vi "User - Filter List.vi"(8 "Error In":errorcluster, 9 "Data to Search":string[](array[string]), 10 "Search From":string[](array[string]), 11 "All List":string[](array[string])) -> (0 "Error Out":errorcluster, 3 "Data Out":string[](array[string]))   [LabVIEW 2020]
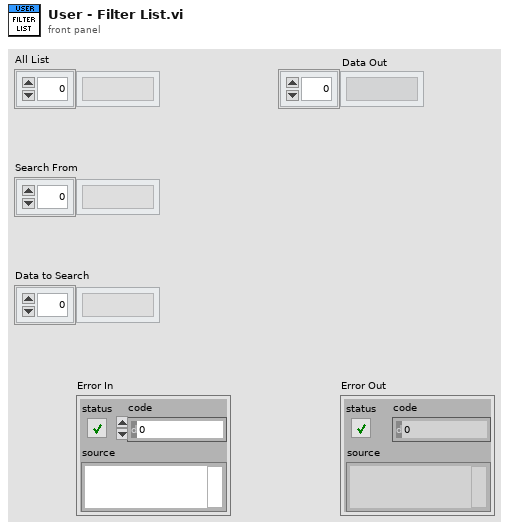
[diagram p1: front panel]
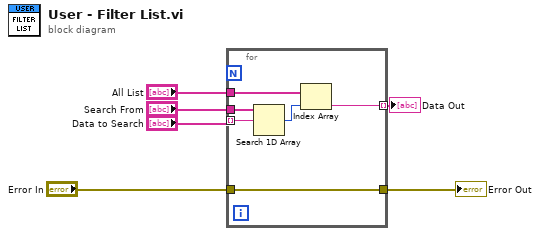
[diagram p0: block diagram]
diagram:
  n1 = for {
    tunnel: "Data to Search" -> [w10] mode=indexing
    tunnel: "All List" -> [w8]
    tunnel: "Search From" -> [w11]
    tunnel: [w7] -> w1 mode=indexing
    tunnel: [w12] -> w6
    tunnel: "Error In" -> [w12]
    n2 = Search 1D Array(1D array=w11, element=w10) -> (index of element=w9:i32)  [unwired: 1 in]
    n3 = Index Array(array=w8, index=w9) -> (element=w7:string)
  }
  "Data Out" <- w1
  "Error Out" <- w6
